vi "Load Data.vi"(8 "error in (no error)":errorcluster) -> (0 "error out":errorcluster, 2 "Sound WAV data":waveform(dbl)[](array[waveform]), 3 "Wind Data":dbl[][](array[numeric]))   [LabVIEW 2018]
uses:
  <vilib>/Utility/file.llb/Read From Spreadsheet File (DBL).vi
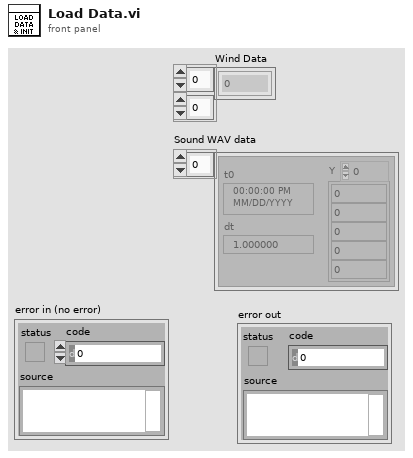
[diagram p1: front panel]
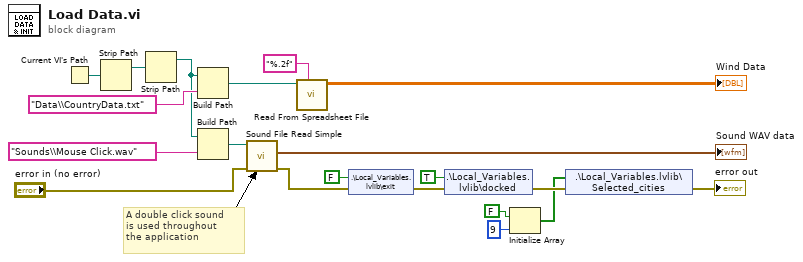
[diagram p0: block diagram]
diagram:
  # "A double click sound\nis used throughout\nthe application"
  n1 = Current VI's Path() -> (path=w12:path)
  n2 = Strip Path(path=w12) -> (stripped path=w18:path)  [unwired: 1 out]
  n3 = Strip Path(path=w18) -> (stripped path=w10:path)  [unwired: 1 out]
  n4 = Build Path(base path=w10, name or relative path="Data\\CountryData.txt") -> (appended path=w14:path)
  n5 = Build Path(base path=w10, name or relative path="Sounds\\Mouse Click.wav") -> (appended path=w19:path)
  n6 = call <vilib>:"Sound File Read Simple.vi"("error in (no error)"="error in (no error)", "path"=w19) -> ("error out"=w8:errorcluster, "data"=→"Sound WAV data":waveform(dbl)[])  [unwired: 6 in, 2 out]
  n7 = call-poly <vilib>:"Read From Spreadsheet File.vi"("format (%.3f)"="%.2f", "file path (dialog if empty)"=w14) -> ("all rows"=→"Wind Data":dbl[][])  [unwired: 5 in, 4 out]
  n8 = shared-variable ".\\Local_Variables.lvlib\\exit"(FALSE ("exit"), error in=w8) -> (error out=w7:errorcluster)
  n9 = shared-variable ".\\Local_Variables.lvlib\\docked"(TRUE ("docked"), error in=w7) -> (error out=w5:errorcluster)
  n10 = Initialize Array(FALSE, 9 ("dimension size")) -> (w3:bool[])
  n11 = shared-variable ".\\Local_Variables.lvlib\\Selected_cities"(w3, error in=w5) -> (error out=→"error out":errorcluster)
